vi "Sound_processing.vi"(0 "Array":waveform(dbl)[](array[waveform]), 5 "Volume":dbl(slide)=1.0 scale=0.0..1.0, 7 "Bass":dbl(slide)=1.0 scale=0.0..1.0, 9 "Mid":dbl(slide)=1.0 scale=0.0..1.0, 11 "Treble":dbl(slide)=1.0 scale=0.0..1.0) -> (4 "Dynamic Data":dynamicdata(waveform), 6 "detected frequencies":dbl[](array[numeric]) format="%.2p", 8 "Power Spectrum / PSD":cluster{"f0":dbl, "df":dbl, "magnitude":dbl[]}[](array[cluster]))   [LabVIEW 2013]
uses:
  <vilib>/measure/matone.llb/Extract Single Tone Information N Chan.vi
  <vilib>/measure/maspectr.llb/FFT Power Spectrum and PSD for N Chan.vi
  <vilib>/measure/NI_MAPro.lvlib
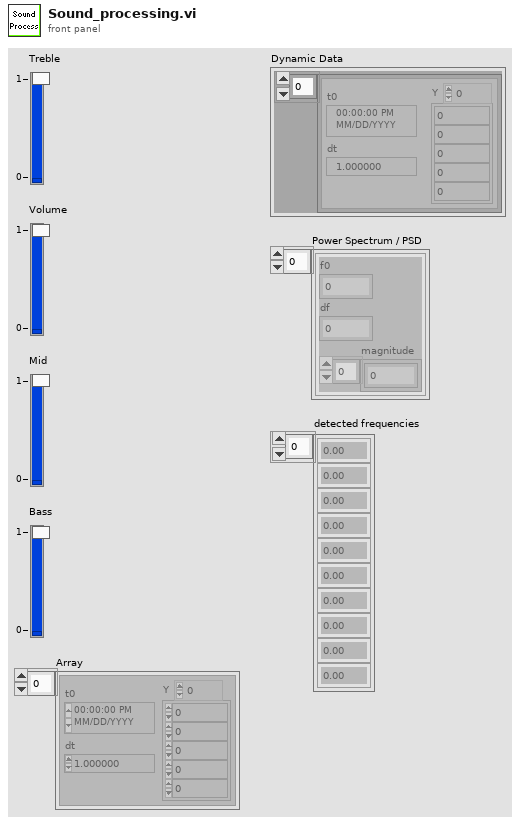
[diagram p1: front panel]
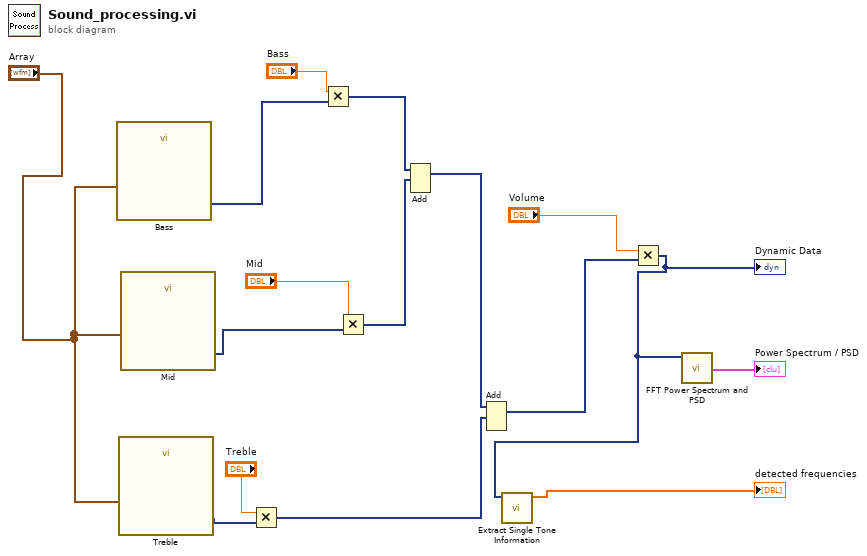
[diagram p0: block diagram]
diagram:
  n1 = call "Bass"("Signal"="Array") -> ("Filtered Signal"=w3:dynamicdata)  [unwired: 9 in, 1 out]
  n2 = call "Treble"("Signal"="Array") -> ("Filtered Signal"=w2:dynamicdata)  [unwired: 9 in, 1 out]
  n3 = call "Mid"("Signal"="Array") -> ("Filtered Signal"=w1:dynamicdata)  [unwired: 9 in, 1 out]
  n4 = Multiply(x="Treble", y=w2) -> (x*y=w6:dynamicdata)
  n5 = Multiply(x="Bass", y=w3) -> (x*y=w4:dynamicdata)
  n6 = Multiply(x="Mid", y=w1) -> (x*y=w5:dynamicdata)
  n7 = Add(1:w5, 2:w4) -> (0:w7:dynamicdata)  [unwired: 1 in, 1 out]
  n8 = Add(1:w6, 2:w7) -> (0:w11:dynamicdata)  [unwired: 1 in, 1 out]
  n9 = Multiply(x="Volume", y=w11) -> (x*y=w15:dynamicdata)
  "Dynamic Data" <- w15
  n10 = call-poly <vilib>:"Extract Single Tone Information.vi"("time signals in"=w15) -> ("detected frequencies"=→"detected frequencies":dbl[])  [unwired: 5 in, 5 out]
  n11 = call-poly <vilib>:"FFT Power Spectrum and PSD.vi"("time signals"=w15) -> ("Power Spectrum / PSD"=→"Power Spectrum / PSD":cluster{"f0":dbl, "df":dbl, "magnitude":dbl[]}[])  [unwired: 7 in, 3 out]
